vi "Init.vi"(8 "error in (no error)":errorcluster, 11 "USD Actor in":refnum<class "USD Actor.lvclass">) -> (0 "error out":errorcluster, 3 "USD Actor out":refnum<class "USD Actor.lvclass">)   [LabVIEW 2020, in "USD Actor.lvlib" / "USD Actor.lvclass"]
uses:
  USD Actor.lvclass
  USD Actor.lvclass/USD Actor.ctl
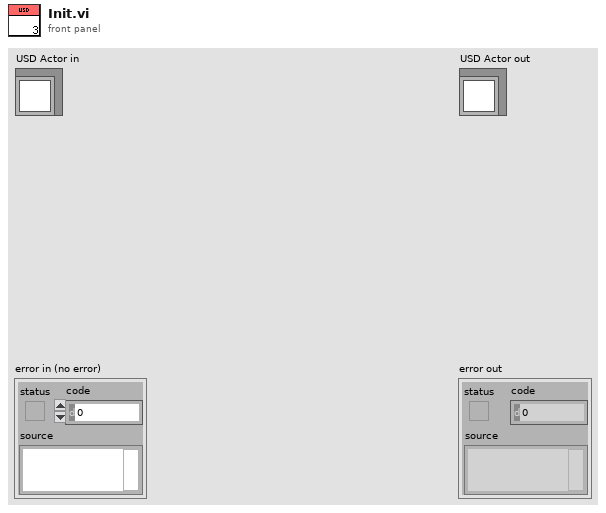
[diagram p1: front panel]
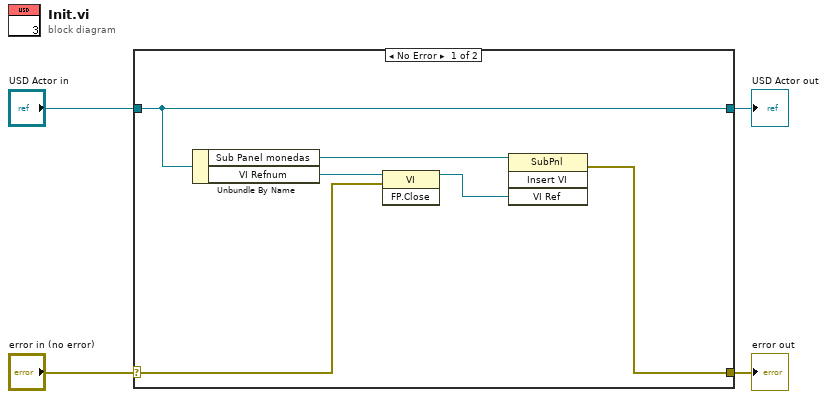
[diagram p0: block diagram]
diagram:
  n1 = case shown="No Error" "error in (no error)" {
    selector: "error in (no error)" -> [w6 w12]
    tunnel: [w5 w12] -> w3
    tunnel: [w7 w11] -> w1
    tunnel: "USD Actor in" -> [w7 w11]
    frame No Error {
      n2 = Unbundle By Name(w7) -> ("Sub Panel monedas"=w10:refnum<vi>, "VI Refnum"=w9:refnum<vi>)
      n3 = invoke class="VI" method="FP.Close"(reference=w9, error in=w6) -> (reference out=w8:refnum<vi>)  [unwired: 1 in, 2 out]
      n4 = invoke class="SubPnl" method="Insert VI"(reference=w10, "VI Ref"=w8) -> (error out=w5:errorcluster)  [unwired: 2 in, 3 out]
    }
    frame Error {
    }
  }
  "error out" <- w3
  "USD Actor out" <- w1
